vi "发送.vi"() -> ()   [LabVIEW 2018]
panel:
  in  "字符串 8":string
  in  "字符串 7":string
  in  "字符串 6":string
  in  "字符串 5":string
  in  "字符串 4":string
  in  "字符串 3":string
  in  "字符串 2":string
  in  "字符串":string
  out "子字符串之后":string
  out "子字符串之前":string
  in  "模拟现场的布尔亮量":bool[](array[boolean])
  out "控制操作信息":string
  out "长度":i32
  out "连接的字符串":string
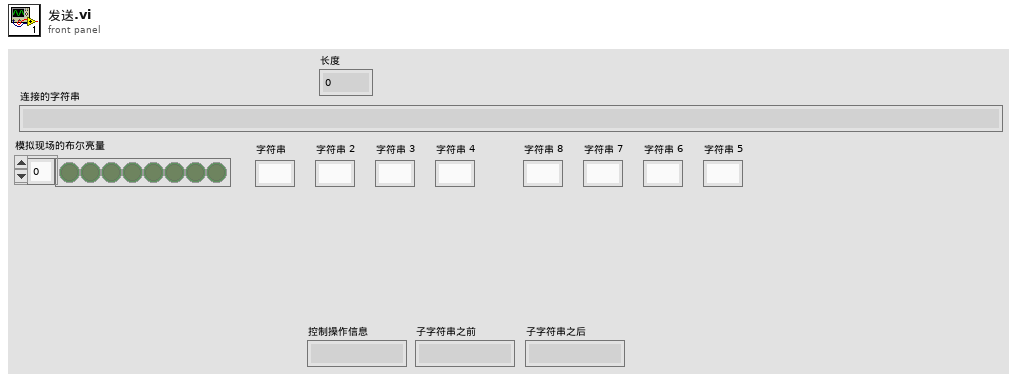
[diagram p1: front panel]
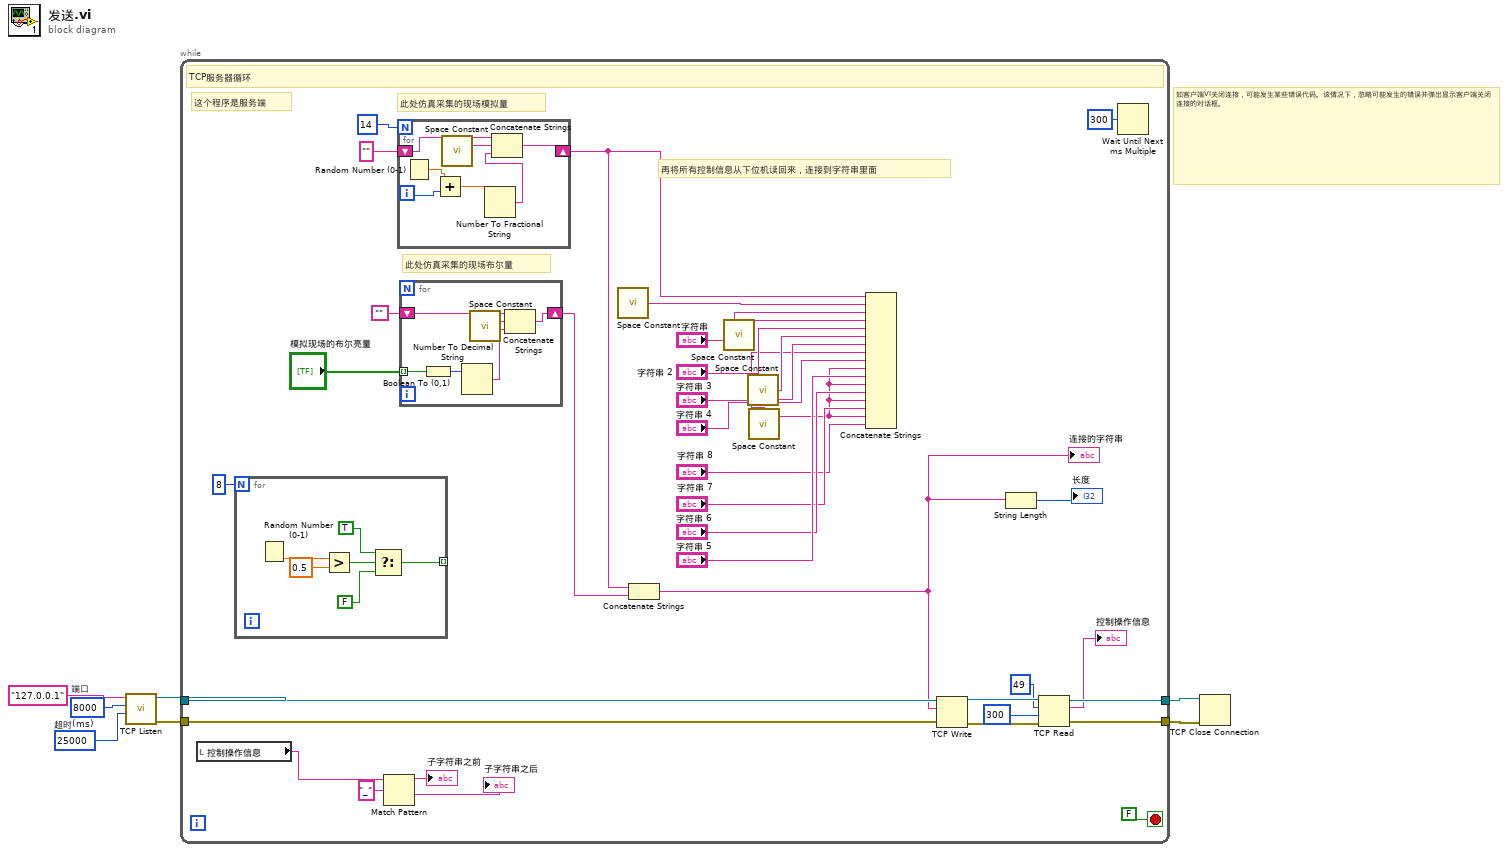
[diagram p0: block diagram]
diagram:
  w4 = u16 8000  # 端口
  w5 = 25000  # 超时(ms)
  # "如客户端VI关闭连接，可能发生某些错误代码。该情况下，忽略可能发生的错误并弹出显示客户端关闭连接的对话框。"
  n1 = call <vilib>:"TCP Listen.vi"("timeout ms (wait forever: -1)"=w5, "port"=w4, "service name"="127.0.0.1") -> ("error out"=w6:errorcluster, "connection ID"=w7:refnum<k5>)  [unwired: 4 in, 3 out]
  n2 = while {
    tunnel: w7 -> [w41]
    tunnel: w6 -> [w40]
    tunnel: [w34] -> w3
    tunnel: [w33] -> w2
    stop <- FALSE stop-if-true
    # "再将所有控制信息从下位机读回来，连接到字符串里面"
    # "此处仿真采集的现场布尔量"
    # "此处仿真采集的现场模拟量"
    # "这个程序是服务端"
    # "TCP服务器循环"
    n3 = local read "控制操作信息"() -> (w28:string)
    n4 = for {
      N: 8 -> [_]
      tunnel: [w44] -> _ mode=indexing
      n5 = Random Number (0-1)() -> (number: 0 to 1=w49:dbl)
      n6 = Greater?(x=w49, y=0.5) -> (0:w47:bool)
      n7 = Select(t=TRUE, s=w47, f=FALSE) -> (s? t:f=w44:bool)
    }
    n8 = Match Pattern(string=w28, regular expression="_" ("正则表达式")) -> (before substring=→"子字符串之前":string, after substring=→"子字符串之后":string)  [unwired: 1 in, 2 out]
    n9 = for {
      N: 14 -> [_]
      shift-right: [w58] -> w11
      shift-left: "" -> [w57]
      i -> [w62]
      n10 = Random Number (0-1)() -> (number: 0 to 1=w61:dbl)
      n11 = Add(x=w61, y=w62) -> (x+y=w60:dbl)
      n12 = call <vilib>:"Space Constant.vi"() -> ("String"=w56:string)
      n13 = Number To Fractional String(number=w60) -> (F-format string=w59:string)  [unwired: 3 in]
      n14 = Concatenate Strings(w57, w56, w59) -> (w58:string)
    }
    n15 = for {
      tunnel: "模拟现场的布尔亮量" -> [w55] mode=indexing
      shift-right: [w50] -> w12
      shift-left: "" -> [w53]
      n16 = Boolean To (0,1)(Boolean=w55) -> (0, 1=w54:i16)
      n17 = Number To Decimal String(number=w54) -> (decimal integer string=w52:string)  [unwired: 1 in]
      n18 = call <vilib>:"Space Constant.vi"() -> ("String"=w51:string)
      n19 = Concatenate Strings(w53, w51, w52) -> (w50:string)
    }
    n20 = call <vilib>:"Space Constant.vi"() -> ("String"=w24:string)
    n21 = Concatenate Strings(w11, w12) -> (w10:string)
    "连接的字符串" <- w10
    n22 = call <vilib>:"Space Constant.vi"() -> ("String"=w22:string)
    n23 = call <vilib>:"Space Constant.vi"() -> ("String"=w20:string)
    n24 = call <vilib>:"Space Constant.vi"() -> ("String"=w14:string)
    n25 = Concatenate Strings(w11, w24, "字符串", w22, "字符串 2", w20, "字符串 3", w14, "字符串 4", w14, "字符串 5", w14, "字符串 6", w14, "字符串 7", w14, "字符串 8") -> ()  [unwired: 1 out]
    n26 = TCP Write(connection ID=w41, data in=w10, error in (no error)=w40) -> (connection ID out=w36:refnum<k5>, error out=w35:errorcluster)  [unwired: 2 out]
    n27 = String Length(string=w10) -> (length=→"长度":i32)
    n28 = TCP Read(connection ID=w36, bytes to read=49 ("读取的字节"), error in (no error)=w35, 9:300 ("超时毫秒(25000)")) -> (connection ID out=w34:refnum<k5>, data out=→"控制操作信息":string, error out=w33:errorcluster)  [unwired: 1 in]
    n29 = Wait Until Next ms Multiple(millisecond multiple=u32 300 ("milliseconds to wait")) -> ()  [unwired: 1 out]
  }
  n30 = TCP Close Connection(connection ID=w3, error in (no error)=w2) -> ()  [unwired: 3 out]
